vi "Image_RAW_Get_Num.vi"(8 "error in (no error)":errorcluster, 11 "RAW refnum In":refnum<file>) -> (0 "error out":errorcluster, 1 "Bytes per Frame":u32, 2 "Total Frame Num":i64, 3 "RAW refnum Out":refnum<file>, 4 "Image Data Config":T1={"Lines of Image Data"=0, "Bytes per Even Line"=0, "Bytes per Odd Line"=0, "Image Data Type"=44, "Total Image Data Block Size"=0, "Image Data Block Offset"=0} {"Image Data Type" format="%x"}, 5 "EBD Config":T2)   [LabVIEW 2020]
uses:
  ctl/Image_EBD_Config.ctl
  ctl/Image_Data_Config.ctl
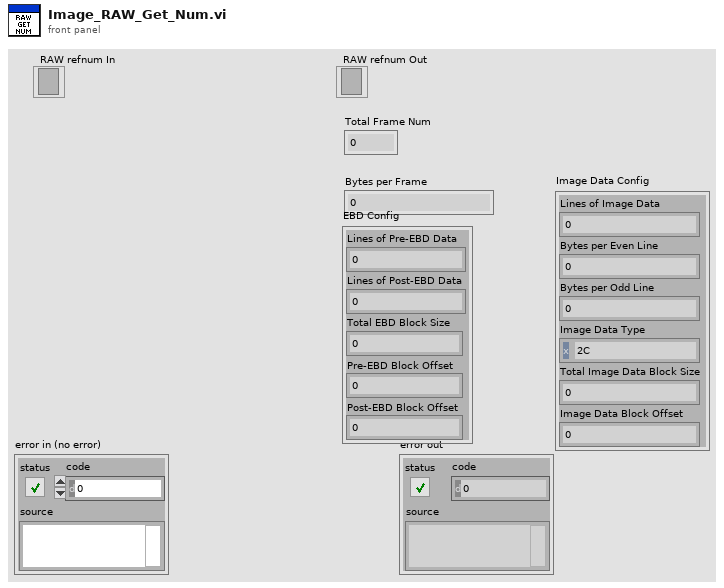
[diagram p1: front panel]
types:
  T1 = typedef "Image_Data_Config.ctl" = cluster{"Lines of Image Data":u16, "Bytes per Even Line":u16, "Bytes per Odd Line":u16, "Image Data Type":u8, "Total Image Data Block Size":u32, "Image Data Block Offset":u32}
  T2 = typedef "Image_EBD_Config.ctl" = cluster{"Lines of Pre-EBD Data":u16, "Lines of Post-EBD Data":u16, "Total EBD Block Size":u32, "Pre-EBD Block Offset ":u32, "Post-EBD Block Offset ":u32}
  T3 = enum16{"big-endian, network order", "native, host order", "little-endian"}
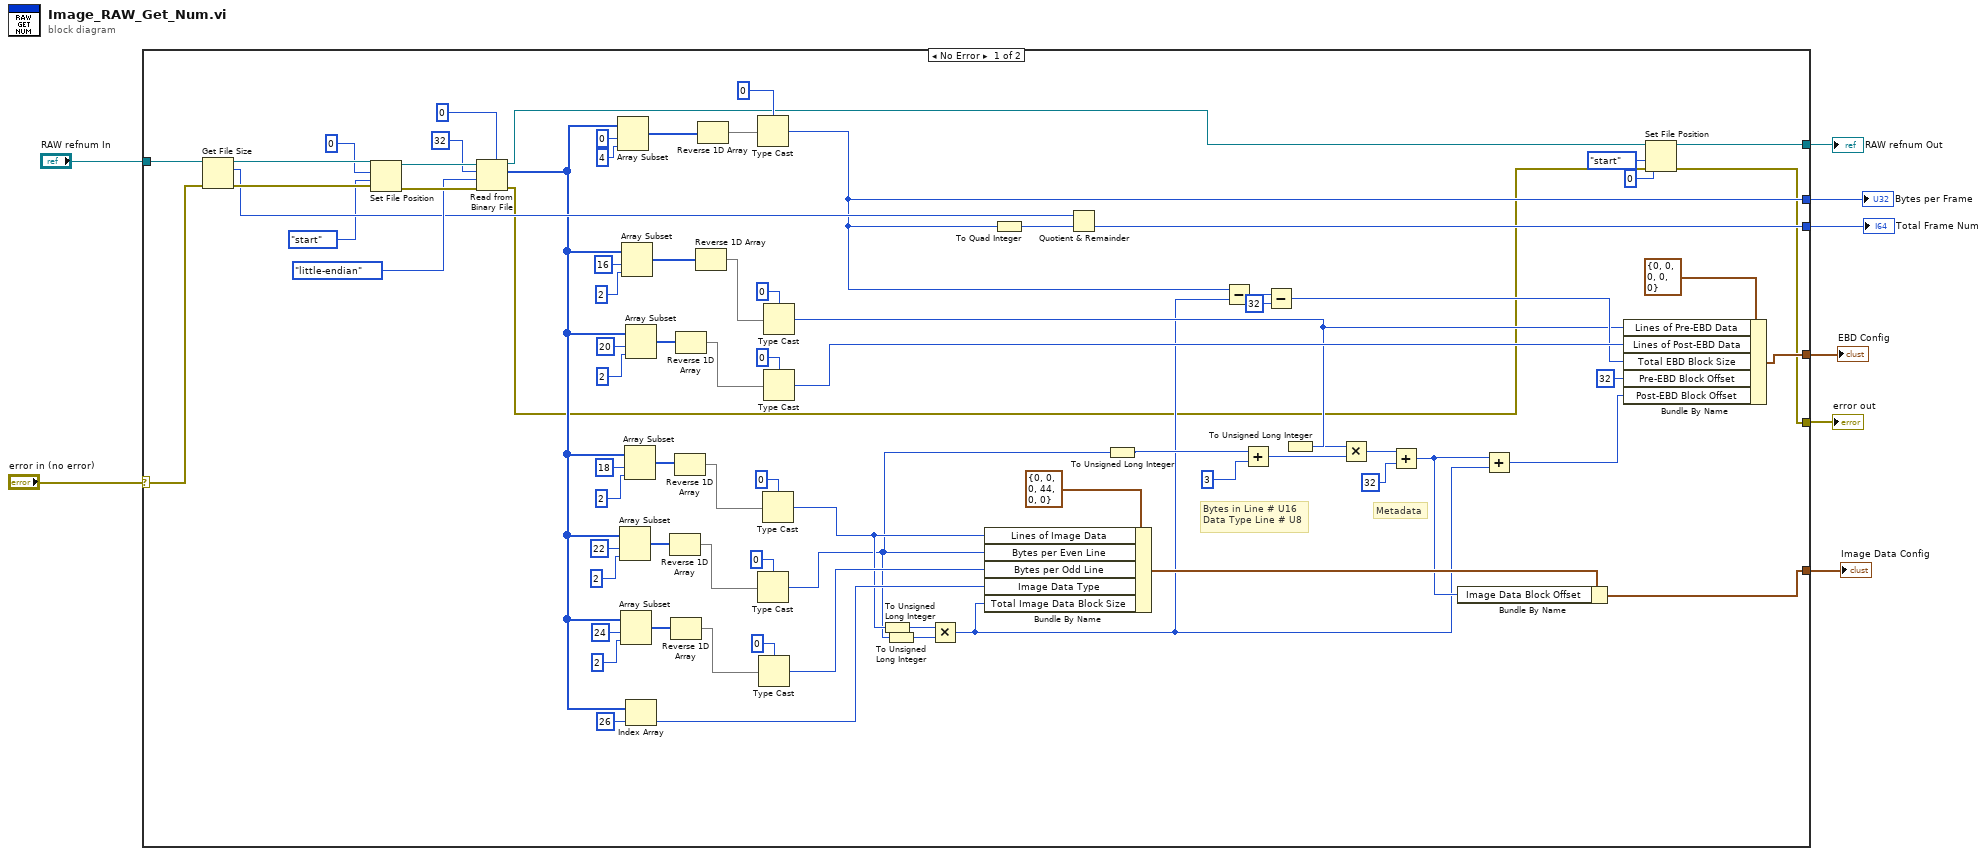
[diagram p0: block diagram]
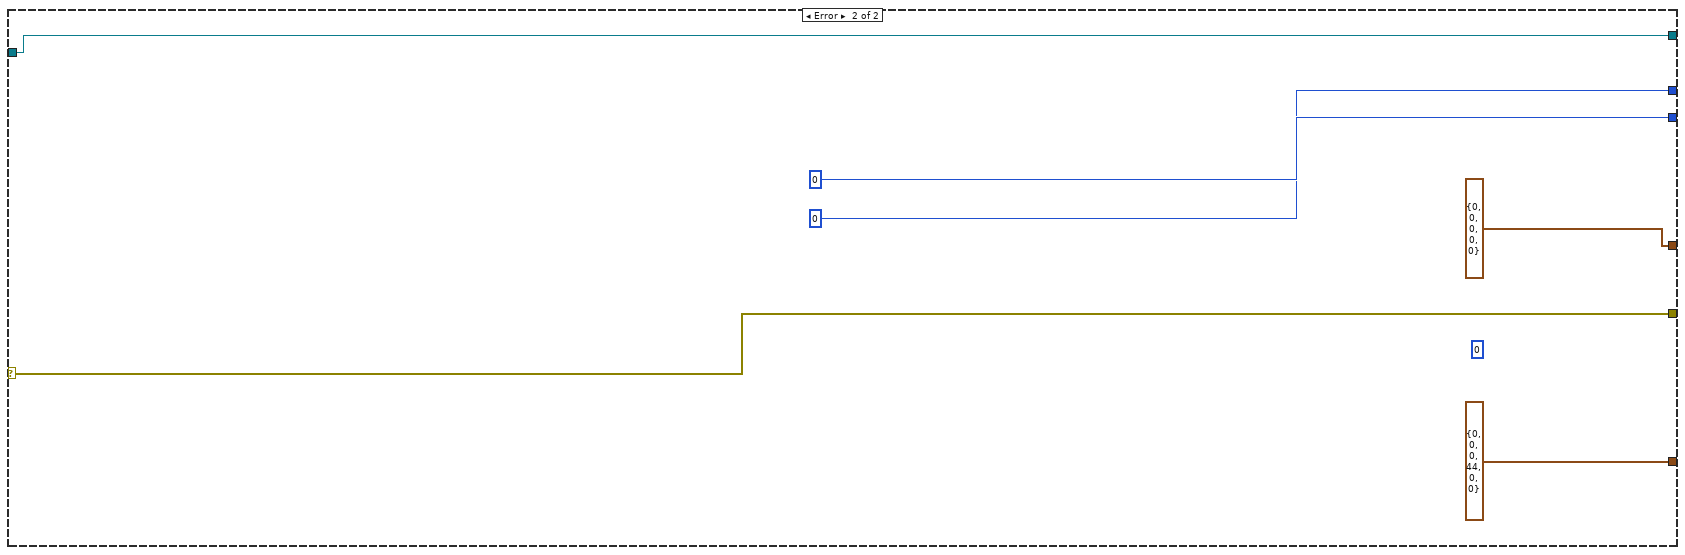
[diagram p2: hidden frame]
diagram:
  n1 = case shown="No Error" "error in (no error)" {
    selector: "error in (no error)" -> [w86 w93]
    tunnel: [w11 w93] -> w7
    tunnel: "RAW refnum In" -> [w87 w92]
    tunnel: [w74 i64 0] -> w5
    tunnel: [w35 u32 0] -> w4
    tunnel: [w13 w92] -> w3
    tunnel: [w16 T2 {"Lines of Pre-EBD Data"=0, "Lines of Post-EBD Data"=0, "Total EBD Block Size"=0, "Pre-EBD Block Offset "=0, "Post-EBD Block Offset "=0} ("EBD Config")] -> w2
    tunnel: [w20 T1 {"Lines of Image Data"=0, "Bytes per Even Line"=0, "Bytes per Odd Line"=0, "Image Data Type"=44, "Total Image Data Block Size"=0, "Image Data Block Offset"=0} ("Image Data Config")] -> w1
    frame No Error {
      # "Metadata"
      # "Bytes in Line # U16\nData Type Line # U8"
      n2 = Get File Size(file=w87, error in=w86) -> (refnum out=w85:refnum<file>, size (in bytes)=w76:i64, 0:w84:errorcluster)
      n3 = Set File Position(offset (in bytes) (0)=i64 0, refnum=w85, from (0:start)=enum16{"start", "end", "current"}."start", error in=w84) -> (refnum out=w82:refnum<file>, error out=w81:errorcluster)
      n4 = Read from Binary File(5:u8 0, 8:w81, 9:T3."little-endian" ("byte order (0:big-endian, network order)"), 10:32 ("count (1)"), 11:w82) -> (0:w12:errorcluster, 2:w39:u8[], 3:w14:refnum<file>)  [unwired: 1 in, 1 out]
      n5 = Array Subset(array=w39, index=0, length=4) -> (w69:u8[])
      n6 = Array Subset(array=w39, index=22, length=2) -> (w52:u8[])
      n7 = Array Subset(array=w39, index=24, length=2) -> (w47:u8[])
      n8 = Array Subset(array=w39, index=16, length=2) -> (w66:u8[])
      n9 = Array Subset(array=w39, index=18, length=2) -> (w41:u8[])
      n10 = Array Subset(array=w39, index=20, length=2) -> (w58:u8[])
      n11 = Index Array(array=w39, index=26) -> (element=w38:u8)
      n12 = Reverse 1D Array(array=w52) -> (reversed array=w54:u8[])
      n13 = Reverse 1D Array(array=w47) -> (reversed array=w49:u8[])
      n14 = Reverse 1D Array(array=w41) -> (reversed array=w43:u8[])
      n15 = Reverse 1D Array(array=w58) -> (reversed array=w60:u8[])
      n16 = Reverse 1D Array(array=w66) -> (reversed array=w65:u8[])
      n17 = Reverse 1D Array(array=w69) -> (reversed array=w73:u8[])
      n18 = Type Cast(type=u32 0, x=w73) -> (*(type *) &x=w35:u32)
      n19 = Type Cast(type=u16 0, x=w54) -> (*(type *) &x=w29:u16)
      n20 = Type Cast(type=u16 0, x=w49) -> (*(type *) &x=w37:u16)
      n21 = Type Cast(type=u16 0, x=w43) -> (*(type *) &x=w36:u16)
      n22 = Type Cast(type=u16 0, x=w65) -> (*(type *) &x=w25:u16)
      n23 = Type Cast(type=u16 0, x=w60) -> (*(type *) &x=w57:u16)
      n24 = To Unsigned Long Integer(number=w36) -> (unsigned 32bit integer=w31:u32)
      n25 = To Unsigned Long Integer(number=w29) -> (unsigned 32bit integer=w30:u32)
      n26 = Multiply(x=w31, y=w30) -> (x*y=w17:u32)
      n27 = Bundle By Name(cluster=T1 {"Lines of Image Data"=0, "Bytes per Even Line"=0, "Bytes per Odd Line"=0, "Image Data Type"=44, "Total Image Data Block Size"=0, "Image Data Block Offset"=0} ("Image Data Config"), "Lines of Image Data"=w36, "Bytes per Even Line"=w29, "Bytes per Odd Line"=w37, "Image Data Type"=w38, "Total Image Data Block Size"=w17) -> (w21:T1)
      n28 = To Quad Integer(1:w35) -> (0:w75:i64)
      n29 = Quotient & Remainder(x=w76, y=w75) -> (floor(x/y)=w74:i64)  [unwired: 1 out]
      n30 = To Unsigned Long Integer(number=w29) -> (unsigned 32bit integer=w27:u32)
      n31 = Subtract(x=w35, y=w17) -> (x-y=w34:u32)
      n32 = Add(x=w27, y=u32 3) -> (x+y=w26:u32)
      n33 = Subtract(x=w34, y=u32 32) -> (x-y=w32:u32)
      n34 = To Unsigned Long Integer(number=w25) -> (unsigned 32bit integer=w24:u32)
      n35 = Multiply(x=w24, y=w26) -> (x*y=w23:u32)
      n36 = Add(x=w23, y=u32 32) -> (x+y=w18:u32)
      n37 = Bundle By Name(cluster=w21, "Image Data Block Offset"=w18) -> (w20:T1)
      n38 = Add(x=w18, y=w17) -> (x+y=w15:u32)
      n39 = Bundle By Name(cluster=T2 {"Lines of Pre-EBD Data"=0, "Lines of Post-EBD Data"=0, "Total EBD Block Size"=0, "Pre-EBD Block Offset "=0, "Post-EBD Block Offset "=0} ("EBD Config"), "Lines of Pre-EBD Data"=w25, "Lines of Post-EBD Data"=w57, "Total EBD Block Size"=w32, "Pre-EBD Block Offset"=u32 32, "Post-EBD Block Offset"=w15) -> (w16:T2)
      n40 = Set File Position(offset (in bytes) (0)=i64 0, refnum=w14, from (0:start)=enum16{"start", "end", "current"}."start", error in=w12) -> (refnum out=w13:refnum<file>, error out=w11:errorcluster)
    }
    frame Error {
      (unwired) u32 0
    }
  }
  "error out" <- w7
  "RAW refnum Out" <- w3
  "Total Frame Num" <- w5
  "Bytes per Frame" <- w4
  "EBD Config" <- w2
  "Image Data Config" <- w1
